vi "Move.vi"(8 "error in (no error)":errorcluster, 10 "Target Position":dbl, 11 "Queue Name":string) -> (0 "error out":errorcluster)   [LabVIEW 2019, in "ADLINK Motion Card.lvlib"]
uses:
  ADLINK Motion Card.lvlib
  Queues/Message Cluster.ctl
  SEQ/SEQ Data.ctl
  Queues/Queues.lvlib
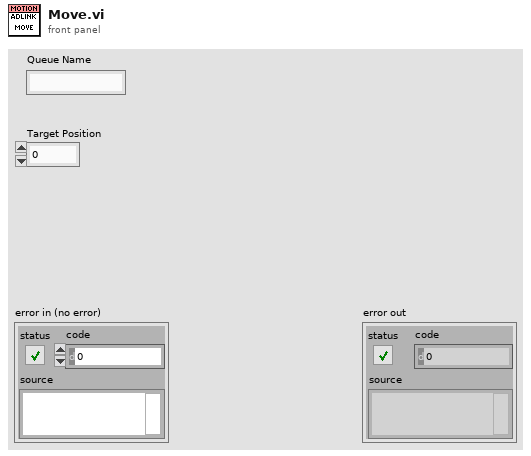
[diagram p1: front panel]
types:
  T1 = typedef "ADLINK Motion Card.lvlib/SEQ Data.ctl" = cluster{"Current Position":dbl, "Target Position":dbl, "Velocity":dbl, "Acceleration":dbl, "Arrived?":bool, "data value reference":refnum<data-value>, "VI Refnum":refnum<vi>}
  T2 = typedef "Queues.lvlib/Message Cluster.ctl" = cluster{"State":string, "Data":variant}
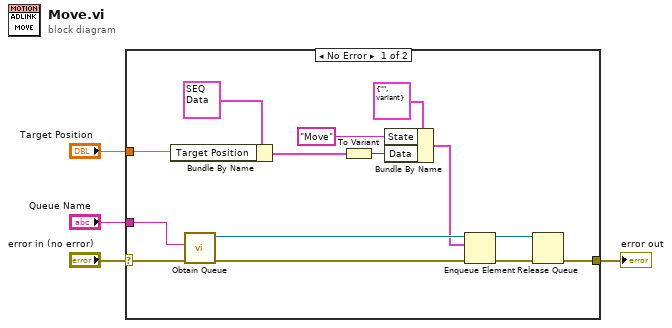
[diagram p0: block diagram]
diagram:
  n1 = case shown="No Error" "error in (no error)" {
    selector: "error in (no error)" -> [w17 w19]
    tunnel: "Queue Name" -> [w18 _]
    tunnel: [w10 w19] -> w2
    tunnel: "Target Position" -> [w5 _]
    frame No Error {
      n2 = Bundle By Name(cluster=T1 {"Current Position"=0.0, "Target Position"=0.0, "Velocity"=0.0, "Acceleration"=0.0, "Arrived?"=FALSE, "data value reference"=refnum, "VI Refnum"=refnum} ("SEQ Data"), "Target Position"=w5) -> (w7:T1)
      n3 = call "Obtain Queue.vi"("Error In"=w17, "Queue Name"=w18) -> ("Error Out"=w16:errorcluster, "queue out"=w15:refnum<queue>)  [unwired: 8 in]
      n4 = To Variant(anything=w7) -> (Variant=w6:variant)
      n5 = Bundle By Name(cluster=T2 {"State"="", "Data"=variant} ("element"), "State"="Move", "Data"=w6) -> (w13:T2)
      n6 = Enqueue Element(queue=w15, element=w13, error in (no error)=w16) -> (queue out=w11:refnum<queue>, error out=w12:errorcluster)  [unwired: 1 in, 1 out]
      n7 = Release Queue(queue=w11, error in (no error)=w12) -> (error out=w10:errorcluster)  [unwired: 1 in, 2 out]
    }
    frame Error {
    }
  }
  "error out" <- w2
